vi "clear_crash.vi"(8 "error in (no error)":errorcluster, 11 "Input":string="34,45,89") -> (0 "error out":errorcluster, 3 "Output":string)   [LabVIEW 2014]
uses:
  <userlib>/Nanonis Prog Interface V5/Nanonis Prog Interface.lvlib
panel:
  out "crashed?":bool
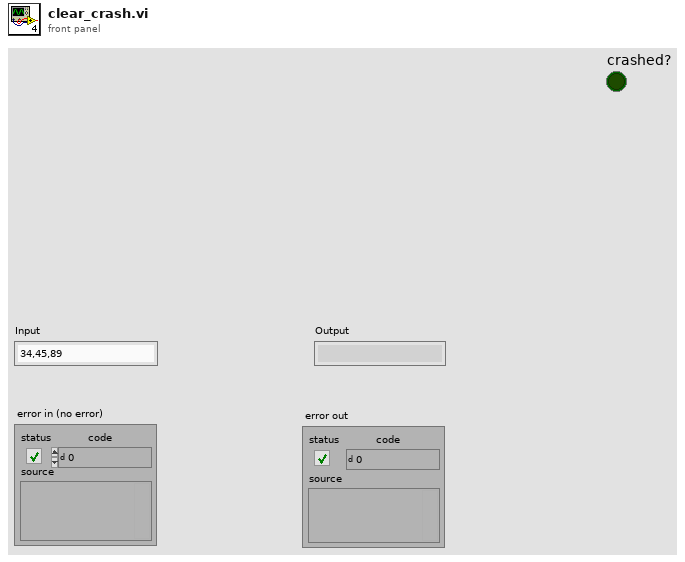
[diagram p1: front panel]
types:
  T1 = enum8{"Group 1", "Group 2", "Group 3", "Group 4", "Group 5", "Group 6"}
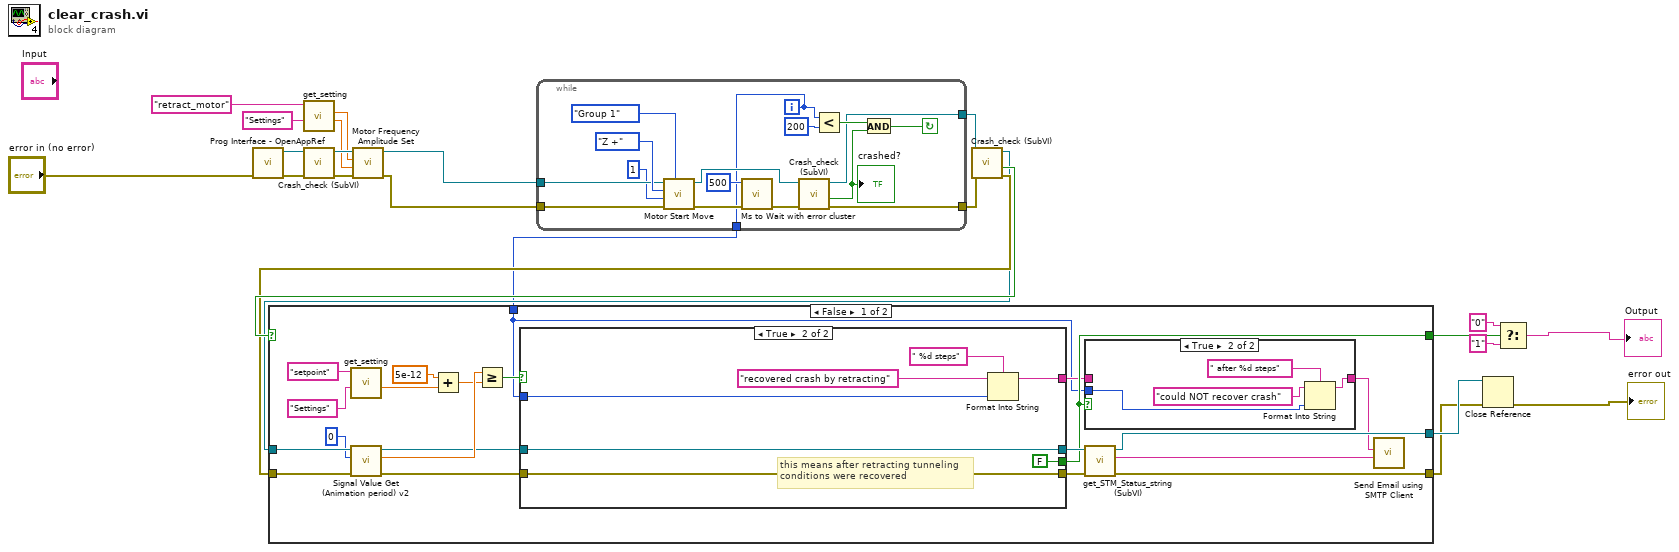
[diagram p0: block diagram]
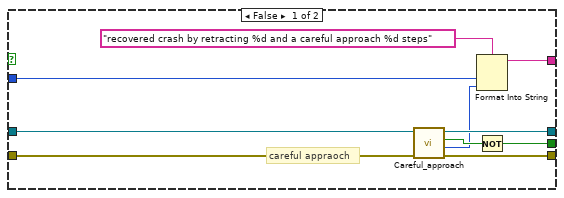
[diagram p3: hidden frame]
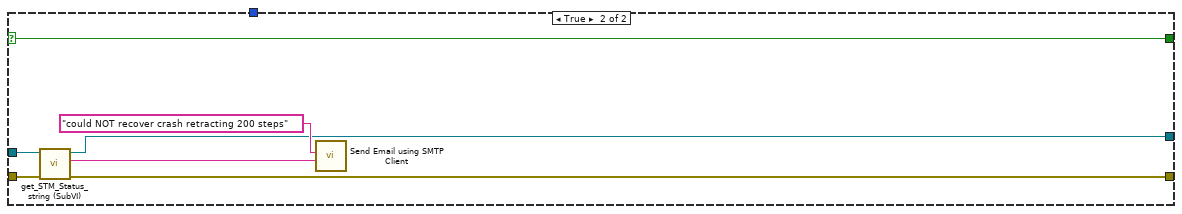
[diagram p4: hidden frame]
diagram:
  n1 = call <userlib>:"Prog Interface - OpenAppRef.vi"("Error in (no error)"="error in (no error)") -> ("Error out"=w20:errorcluster, "Application reference"=w21:refnum<vi>)  [unwired: 5 in]
  n2 = call "get_setting.vi"("section"="Settings", "key"="retract_motor") -> ("output 2"=w12:dbl, "output 1"=w13:dbl)  [unwired: 5 in, 3 out]
  n3 = call "Crash_check (SubVI).vi"("error in (no error)"=w20, "Application in"=w21) -> ("error out"=w15:errorcluster, "Application out"=w14:refnum<vi>)  [unwired: 7 in, 1 out]
  n4 = call <userlib>:"Motor Frequency Amplitude Set.vi"("Error in (no error)"=w15, "Amplitude (V) (NaN=no change)"=w12, "Frequency (Hz) (NaN=no change)"=w13, "Application ref in"=w14) -> ("Error out"=w10:errorcluster, "Application ref out"=w11:refnum<vi>)  [unwired: 6 in]
  n5 = while {
    tunnel: w11 -> [w38]
    tunnel: w10 -> [w37]
    tunnel: [w27] -> w9
    tunnel: [w26] -> w8
    tunnel: [w25] -> w1
    i -> [w25]
    stop <- w29 continue-if-true
    n6 = call <userlib>:"Motor Start Move.vi"("Group"=T1."Group 1", "Error in (no error)"=w37, "Number of steps"=u16 1, "Direction"=enum16{"X +", "X -", "Y +", "Y -", "Z +", "Z -"}."Z +", "Application ref in"=w38) -> ("Error out"=w33:errorcluster, "Application ref out"=w35:refnum<vi>)  [unwired: 4 in]
    n7 = call <userlib>:"Ms to Wait with error cluster.vi"("error in (no error)"=w33, "milliseconds to wait"=u32 500) -> ("error out"=w32:errorcluster)  [unwired: 4 in, 1 out]
    n8 = call "Crash_check (SubVI).vi"("error in (no error)"=w32, "Application in"=w35) -> ("error out"=w27:errorcluster, "crashed?"=w34:bool, "Application out"=w26:refnum<vi>)  [unwired: 7 in]
    "crashed?" <- w34
    n9 = Less?(x=w25, y=200) -> (x < y?=w28:bool)
    n10 = And(x=w28, y=w34) -> (x .and. y?=w29:bool)
  }
  n11 = call "Crash_check (SubVI).vi"("error in (no error)"=w9, "Application in"=w8) -> ("error out"=w6:errorcluster, "crashed?"=w7:bool, "Application out"=w5:refnum<vi>)  [unwired: 7 in]
  n12 = case shown="False" w7 {
    selector: w7 -> [_ w90]
    tunnel: w6 -> [w59 w86]
    tunnel: w5 -> [w58 w88]
    tunnel: [w43 w90] -> w4
    tunnel: [w48 w87] -> w3
    tunnel: [w46 w85] -> w2
    tunnel: w1 -> [w41 _]
    frame False {
      n13 = call "get_setting.vi"("section"="Settings", "key"="setpoint") -> ("output 2"=w55:dbl)  [unwired: 5 in, 4 out]
      n14 = call <userlib>:"Signal Value Get (Animation period) v2.vi"("error in (no error)"=w59, "Signal index (0-79)"=i8 0, "Application ref in"=w58) -> ("error out"=w50:errorcluster, "Signal value"=w56:sgl, "Application ref out"=w51:refnum<vi>)  [unwired: 5 in]
      n15 = Add(x=5e-12, y=w55) -> (x+y=w54:dbl)
      n16 = Greater Or Equal?(x=w56, y=w54) -> (x >= y?=w52:bool)
      n17 = case shown="True" w52 {
        tunnel: [w71 FALSE] -> w43
        tunnel: w51 -> [w76 w81]
        tunnel: w50 -> [w75 w82]
        tunnel: [w74 w81] -> w49
        tunnel: [w73 w82] -> w47
        tunnel: [w70 w79] -> w42
        tunnel: w41 -> [w68 w78]
        frame False {
          # "careful appraoch"
          n18 = call "Careful_approach.vi"("Error in (no error)"=w75, "Application ref in"=w76) -> ("Error out"=w73:errorcluster, "steps_taken"=w67:i32, "approached?"=w72:bool, "Application ref out"=w74:refnum<vi>)  [unwired: 6 in]
          n19 = Format Into String(format string="recovered crash by retracting %d and a careful approach %d steps" ("Subject"), w68, w67) -> (resulting string=w70:string)  [unwired: 2 in, 1 out]
          n20 = Not(x=w72) -> (.not. x?=w71:bool)
        }
        frame True {
          # "this means after retracting tunneling\nconditions were recovered"
          n21 = Format Into String(format string=" %d steps", initial string="recovered crash by retracting" ("Subject"), w78) -> (resulting string=w79:string)  [unwired: 1 in, 1 out]
        }
      }
      n22 = case shown="True" w43 {
        tunnel: [w62 w65] -> w44
        tunnel: w42 -> [w62 _]
        tunnel: w41 -> [_ w64]
        frame False {
        }
        frame True {
          n23 = Format Into String(format string=" after %d steps", initial string="could NOT recover crash" ("Subject"), w64) -> (resulting string=w65:string)  [unwired: 1 in, 1 out]
        }
      }
      n24 = call "get_STM_Status_string (SubVI).vi"("error in (no error)"=w47, "Application in"=w49) -> ("error out"=w46:errorcluster, "JSON string"=w45:string, "Application out"=w48:refnum<vi>)  [unwired: 7 in]
      n25 = call "Send Email using SMTP Client.vi"("Message"=w45, "subject"=w44) -> ()  [unwired: 9 in, 1 out]
    }
    frame True {
      n26 = call "get_STM_Status_string (SubVI).vi"("error in (no error)"=w86, "Application in"=w88) -> ("error out"=w85:errorcluster, "JSON string"=w84:string, "Application out"=w87:refnum<vi>)  [unwired: 7 in]
      n27 = call "Send Email using SMTP Client.vi"("Message"=w84, "subject"="could NOT recover crash retracting 200 steps" ("Subject")) -> ()  [unwired: 9 in, 1 out]
    }
  }
  n28 = Close Reference(reference=w3, error in (no error)=w2) -> (error out=→"error out":errorcluster)
  n29 = Select(t="0", s=w4, f="1") -> (s? t:f=→"Output":string)
